vi "Write TestApplication.vi"(8 "error in (no error)":errorcluster, 10 "TestApplication":refnum<class "TestApplication.lvclass">, 11 "TestApplicationError in":refnum<class "TestApplicationError.lvclass">) -> (0 "error out":errorcluster, 3 "TestApplicationError out":refnum<class "TestApplicationError.lvclass">)   [LabVIEW 2022 SP3, in "Demo.lvlib" / "TestApplicationError.lvclass"]
uses:
  TestApplicationError.lvclass
  TestApplication/TestApplication.lvclass
  TestApplicationError.lvclass/TestApplicationError.ctl
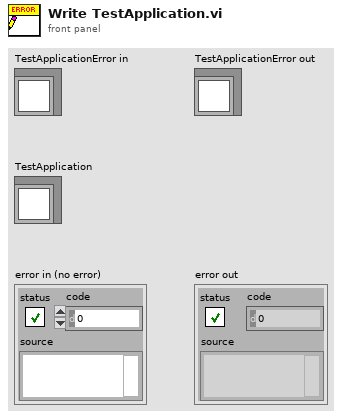
[diagram p1: front panel]
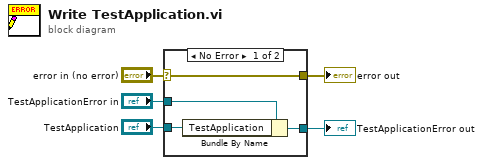
[diagram p0: block diagram]
diagram:
  n1 = case shown="No Error" "error in (no error)" {
    selector: "error in (no error)" -> [w9 w10]
    tunnel: [w9 w10] -> w4
    tunnel: [w7 w11] -> w2
    tunnel: "TestApplicationError in" -> [w8 w11]
    tunnel: "TestApplication" -> [w6 _]
    frame No Error {
      n2 = Bundle By Name(cluster=w8, "TestApplication"=w6) -> (w7:refnum<class "TestApplicationError.lvclass">)
    }
    frame Error {
    }
  }
  "error out" <- w4
  "TestApplicationError out" <- w2
